vi "dsyr2 - Symmetric Matrix Rank-2 Update (DBL).vi"(6 "alpha":dbl=1.0, 8 "matrix A type":T1=3 items=["Lower Triangular"=2, "Upper Triangular"=3], 9 "A":T2, 10 "y":dbl[](array[numeric]), 11 "x":dbl[](array[numeric])) -> (0 "error":i32, 3 "dsyr2":T2)   [LabVIEW 2014, in "NI_AALBLAS.lvlib"]
doc: "Calculates the rank-2 update of the upper or lower triangular component of a symmetric matrix."
uses:
  NI_AALBLAS.lvlib
  RealMatrix.ctl
  LV_UpLo.ctl
  Fucntion.ctl
  Order.ctl
  BLAS2 Utility(DBL).vi
  NI_Matrix.lvlib
panel:
  # "dsyr2=alpha*x*y'+alpha*y*x'+A"
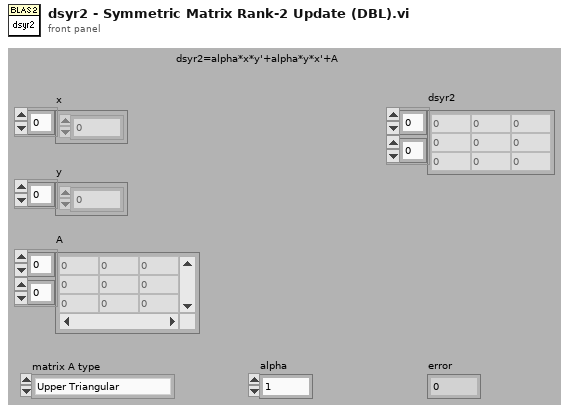
[diagram p1: front panel]
types:
  T1 = typedef "NI_AALBLAS.lvlib/LV_UpLo.ctl" = i32
  T2 = typedef "NI_Matrix.lvlib/RealMatrix.ctl" = dbl[][]
  T3 = typedef "NI_AALBLAS.lvlib/Order.ctl" = i32
  T4 = typedef "NI_AALBLAS.lvlib/Fucntion.ctl" = u16
  T5 = typedef "NI_AALBLAS.lvlib/UpLo.ctl" = i32
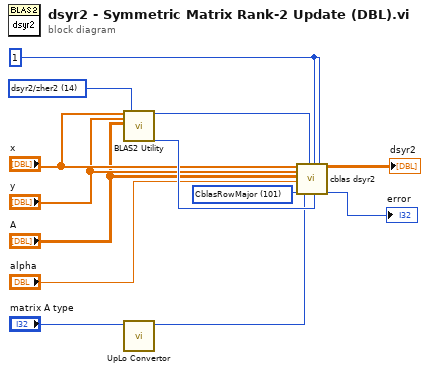
[diagram p0: block diagram]
diagram:
  w1 = 1 ("incX")
  w2 = T3 101 items=["CblasRowMajor"=101, "CblasColMajor"=102] ("order")
  w4 = T4 14 items=["ddot/zdotu/zdotc", "daxpy/zaxpy", "dnrm2/dznrm2", "dasum/dzasum", "dcopy/zcopy", "dswap/zswap", "drotm", "drot/zdrot", "idamax/izamax", "idamin/izamin", "dgemv/zgemv", "dsymv/zhemv", "dtrmv/ztrmv", "dsyr/zher", "dsyr2/zher2", "dger/zgeru/zgerc", "dtrsv/ztrsv", "dgemm/zgemm", "dsymm/zsymm/zhemm", "dtrmm/ztrmm", "dsyrk/zsyrk/zherk", "dsyr2k/zsyr2k/zher2k", "dtrsm/ztrsm"] ("function")
  n1 = call-poly "BLAS2 Utility.vi"("x"="x", "y"="y", "A"="A", "function"=w4) -> ("lda"=w3:i32, "n"=w13:i32)  [unwired: 1 in, 13 out]
  n2 = call "UpLo Convertor.vi"("triangle matrix type"="matrix A type") -> ("uplo"=w10:T5)  [unwired: 10 out]
  n3 = call "cblas dsyr2.vi"("x"="x", "y"="y", "A"="A", "alpha"="alpha", "order"=w2, "uplo"=w10, "lda"=w3, "incx"=w1, "n"=w13, "incy"=w1) -> ("dsyr2"=→"dsyr2":T2, "error"=→"error":i32)  [unwired: 8 out]
